vi "cumplimiento.vi"(8 "error in (no error)":errorcluster, 11 "Prueba06 in":refnum<class "Prueba06.lvclass">) -> (0 "error out":errorcluster, 3 "Prueba06 out":refnum<class "Prueba06.lvclass">)   [LabVIEW 2019, in "Prueba06.lvclass"]
uses:
  Prueba06.lvclass
  Prueba06.lvclass/Prueba06.ctl
panel:
  out "cumpimiento":string
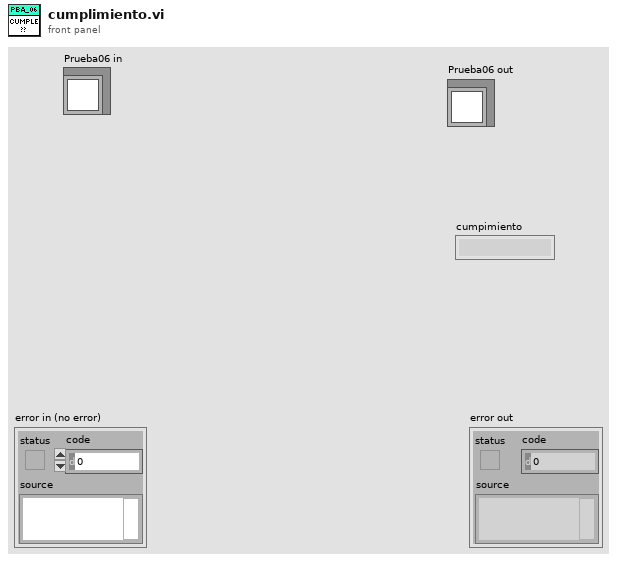
[diagram p1: front panel]
types:
  T1 = cluster{"Medido":dbl, "Error":dbl, "Ref":dbl, "Incert_exp":dbl, "Tol+":dbl, "Tol-":dbl, "fila":i32}
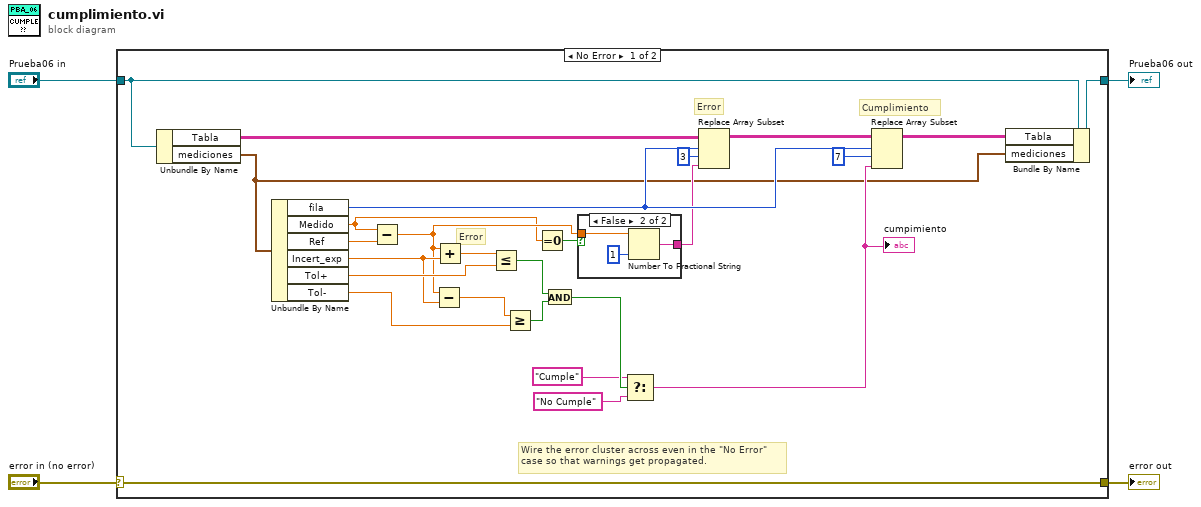
[diagram p0: block diagram]
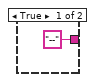
[diagram p2: hidden frame]
diagram:
  n1 = case shown="No Error" "error in (no error)" {
    selector: "error in (no error)" -> [w30 w36]
    tunnel: [w30 w36] -> w3
    tunnel: [w9 w35] -> w2
    tunnel: "Prueba06 in" -> [w7 w35]
    frame No Error {
      # "Cumplimiento"
      # "Error"
      # "Error"
      # "Wire the error cluster across even in the \"No Error\"\ncase so that warnings get propagated."
      n2 = Unbundle By Name(w7) -> ("Tabla"=w6:string[][], "mediciones"=w5:T1)
      n3 = Unbundle By Name(w5) -> ("fila"=w15:i32, "Medido"=w10:dbl, "Ref"=w22:dbl, "Incert_exp"=w20:dbl, "Tol+"=w21:dbl, "Tol-"=w19:dbl)
      n4 = Subtract(x=w10, y=w22) -> (x-y=w11:dbl)
      n5 = Subtract(x=w11, y=w20) -> (x-y=w26:dbl)
      n6 = Add(x=w11, y=w20) -> (x+y=w29:dbl)
      n7 = Less Or Equal?(x=w29, y=w21) -> (x <= y?=w28:bool)
      n8 = Greater Or Equal?(x=w26, y=w19) -> (x >= y?=w27:bool)
      n9 = Equal To 0?(x=w10) -> (x = 0?=w12:bool)
      n10 = And(x=w28, y=w27) -> (x .and. y?=w25:bool)
      n11 = case shown="False" w12 {
        tunnel: w11 -> [_ w34]
        tunnel: ["--" w32] -> w13
        frame True {
        }
        frame False {
          n12 = Number To Fractional String(number=w34, precision (6)=i16 1) -> (F-format string=w32:string)  [unwired: 2 in]
        }
      }
      n13 = Select(t="Cumple", s=w25, f="No Cumple") -> (s? t:f=w18:string)
      "cumpimiento" <- w18
      n14 = Replace Array Subset(array=w6, new element=w13, index (row)=w15, index (col)=3 ("disabled index (col)")) -> (w16:string[][])
      n15 = Replace Array Subset(array=w16, new element=w18, index (row)=w15, index (col)=7 ("index (row)")) -> (w8:string[][])
      n16 = Bundle By Name(cluster=w7, "Tabla"=w8, "mediciones"=w5) -> (w9:refnum<class "Prueba06.lvclass">)
    }
    frame Error {
    }
  }
  "error out" <- w3
  "Prueba06 out" <- w2
